vi "Fetch Acquired Data (U64).vi"(5 "FIFO Type":T1, 7 "Timeout (s)":i32=5, 8 "error out":errorcluster, 9 "Swap?":bool, 10 "Samples":i32=-1, 11 "FPGA Reference In":refnum<k20>) -> (0 "error out":errorcluster, 2 "Data":u64[](array[numeric]), 3 "FPGA Reference Out":refnum<k20>, 4 "Elements Remaining":u32)   [LabVIEW 2012, in "FlexRIO Host Library (User).lvlib"]
uses:
  <userlib>/FlexRIO Host Library/FlexRIO Host API/Acquire/FIFO Type.ctl
  <vilib>/Utility/error.llb/Error Cluster From Error Code.vi
  <vilib>/rvi/errors/niLvFpgaAdjustHostInterfaceError.vi
  <vilib>/rvi/interface/nirviMethod/nirviMethod.xnode
  <userlib>/FlexRIO Host Library/FlexRIO Host Library (User).lvlib
  <vilib>/rvi/errors/niLvFpgaMergeErrorWithErrorCode.vi
  <vilib>/FPGAPlugInAG/Dynamic/niLvFpga_ReadFifo_Dynamic.vi
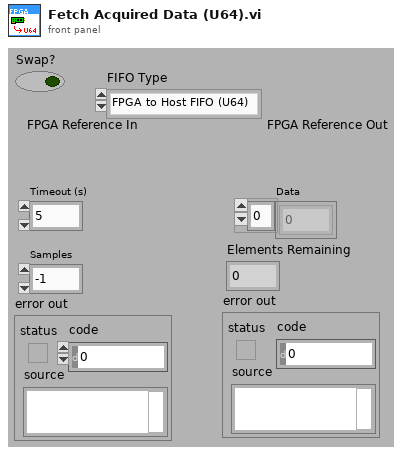
[diagram p1: front panel]
types:
  T1 = typedef "FIFO Type.ctl" = enum16{"FPGA to Host FIFO (U64)", "Generic", "FPGA to Host FIFO (U32)", "Fast FIFO"}
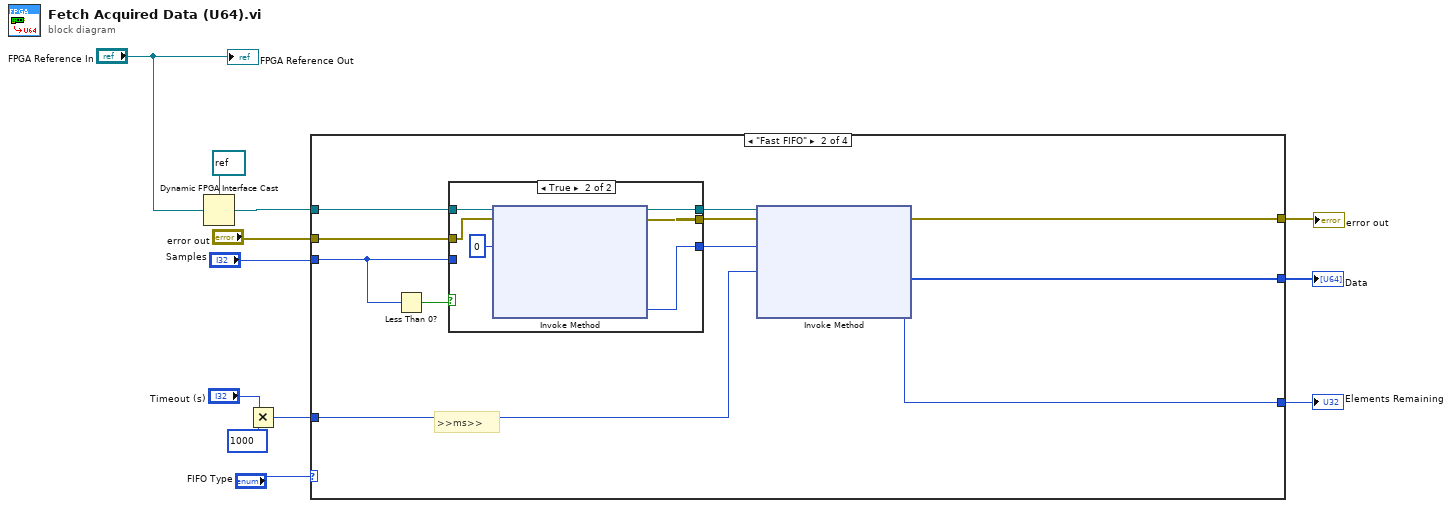
[diagram p0: block diagram]
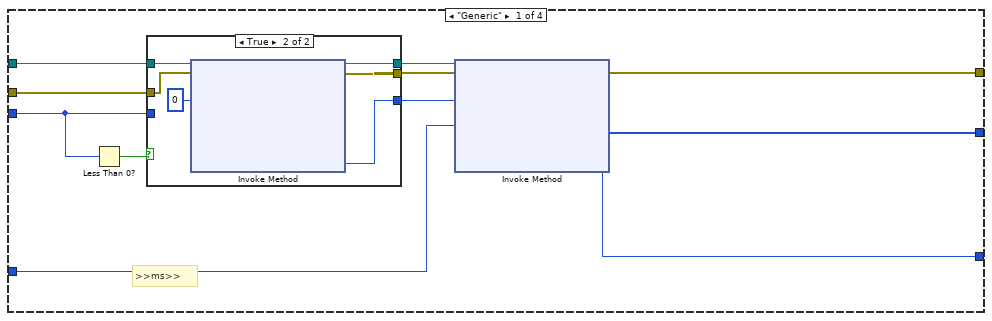
[diagram p2: hidden frame]
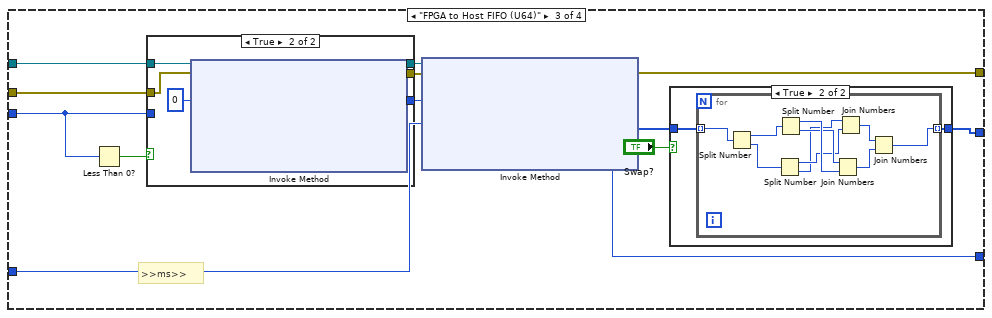
[diagram p5: hidden frame]
diagram:
  n1 = Dynamic FPGA Interface Cast(Session In=refnum<k20> refnum ("Type"), Type="FPGA Reference In") -> (Session Out=w10:refnum<k20>)
  n2 = Multiply(x="Timeout (s)", y=1000) -> (x*y=w3:i32)
  n3 = case shown="\"Fast FIFO\"" "FIFO Type" {
    tunnel: [w19 w39 w54 _] -> w12
    tunnel: w10 -> [w18 w38 w61 _]
    tunnel: [w17 w37 w60 w88] -> w9
    tunnel: [w16 w36 w59 _] -> w8
    tunnel: "error out" -> [w14 w34 w58 w88]
    tunnel: "Samples" -> [w13 w33 w57 _]
    tunnel: w3 -> [w15 w35 w56 _]
    frame "Generic" {
      # ">>ms>>"
      n4 = Less Than 0?(x=w13) -> (x < 0?=w23:bool)
      n5 = case shown="True" w23 {
        tunnel: w18 -> [w26 w32]
        tunnel: w14 -> [w25 w31]
        tunnel: [w26 w30] -> w22
        tunnel: [w25 w29] -> w21
        tunnel: [w24 w28] -> w20
        tunnel: w13 -> [w24 _]
        frame False {
        }
        frame True {
          n6 = xnode "Invoke Method"("FPGA VI Reference In"=w32, "error in"=w31, "Number of Elements"=u32 0) -> ("FPGA VI Reference Out"=w30:refnum<k20>, "error out"=w29:errorcluster, "Elements Remaining"=w28:u32)  [unwired: 1 in, 1 out]
        }
      }
      n7 = xnode "Invoke Method"("FPGA VI Reference In"=w22, "error in"=w21, "Number of Elements"=w20, "Timeout (ms)"=w15) -> ("error out"=w17:errorcluster, "Data"=w19:u64[], "Elements Remaining"=w16:u32)  [unwired: 1 out]
    }
    frame "Fast FIFO" {
      # ">>ms>>"
      n8 = Less Than 0?(x=w33) -> (x < 0?=w43:bool)
      n9 = case shown="True" w43 {
        tunnel: w38 -> [w46 w52]
        tunnel: w34 -> [w45 w51]
        tunnel: [w46 w50] -> w42
        tunnel: [w45 w49] -> w41
        tunnel: [w44 w48] -> w40
        tunnel: w33 -> [w44 _]
        frame False {
        }
        frame True {
          n10 = xnode "Invoke Method"("FPGA VI Reference In"=w52, "error in"=w51, "Number of Elements"=u32 0) -> ("FPGA VI Reference Out"=w50:refnum<k20>, "error out"=w49:errorcluster, "Elements Remaining"=w48:u32)  [unwired: 1 in, 1 out]
        }
      }
      n11 = xnode "Invoke Method"("FPGA VI Reference In"=w42, "error in"=w41, "Number of Elements"=w40, "Timeout (ms)"=w35) -> ("error out"=w37:errorcluster, "Data"=w39:u64[], "Elements Remaining"=w36:u32)  [unwired: 1 out]
    }
    frame "FPGA to Host FIFO (U64)" {
      # ">>ms>>"
      n12 = Less Than 0?(x=w57) -> (x < 0?=w65:bool)
      n13 = case shown="True" w65 {
        tunnel: w61 -> [w81 w87]
        tunnel: w58 -> [w80 w86]
        tunnel: [w81 w85] -> w64
        tunnel: [w80 w84] -> w63
        tunnel: [w79 w83] -> w62
        tunnel: w57 -> [w79 _]
        frame False {
        }
        frame True {
          n14 = xnode "Invoke Method"("FPGA VI Reference In"=w87, "error in"=w86, "Number of Elements"=u32 0) -> ("FPGA VI Reference Out"=w85:refnum<k20>, "error out"=w84:errorcluster, "Elements Remaining"=w83:u32)  [unwired: 1 in, 1 out]
        }
      }
      n15 = xnode "Invoke Method"("FPGA VI Reference In"=w64, "error in"=w63, "Number of Elements"=w62, "Timeout (ms)"=w56) -> ("error out"=w60:errorcluster, "Data"=w55:u64[], "Elements Remaining"=w59:u32)  [unwired: 1 out]
      n16 = case shown="True" "Swap?" {
        tunnel: w55 -> [w66 w68]
        tunnel: [w66 w67] -> w54
        frame False {
        }
        frame True {
          n17 = for {
            tunnel: w68 -> [w78] mode=indexing
            tunnel: [w69] -> w67 mode=indexing
            n18 = Split Number(x=w78) -> (hi(x)=w76:u32, lo(x)=w77:u32)
            n19 = Split Number(x=w77) -> (hi(x)=w73:u16, lo(x)=w72:u16)
            n20 = Split Number(x=w76) -> (hi(x)=w75:u16, lo(x)=w74:u16)
            n21 = Join Numbers(hi=w74, lo=w75) -> ((hi.lo)=w70:u32)
            n22 = Join Numbers(hi=w72, lo=w73) -> ((hi.lo)=w71:u32)
            n23 = Join Numbers(hi=w71, lo=w70) -> ((hi.lo)=w69:u64)
          }
        }
      }
    }
    frame "FPGA to Host FIFO (U32)" {
    }
  }
  "Data" <- w12
  "error out" <- w9
  "Elements Remaining" <- w8
  "FPGA Reference Out" <- "FPGA Reference In"
